vi "Supported .NET colors.vi"() -> (0 "Color Names":T1[](array[typedef]), 2 "Colors":u32[](array[numeric]))   [LabVIEW 2021, in "Rich Text Box.lvlib"]
uses:
  Rich Text Box.lvlib
  Text Colors.ctl
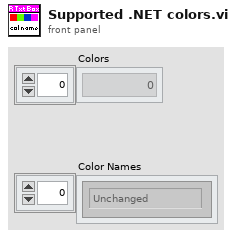
[diagram p1: front panel]
types:
  T1 = typedef "Rich Text Box.lvlib/Text Colors.ctl" = enum16{"Unchanged", "Black", "Blue", "Cyan", "Maroon", "Gray", "Violet", "Green", "Light Green", "Orange", "Yellow", "Magenta", "Red", "White"}
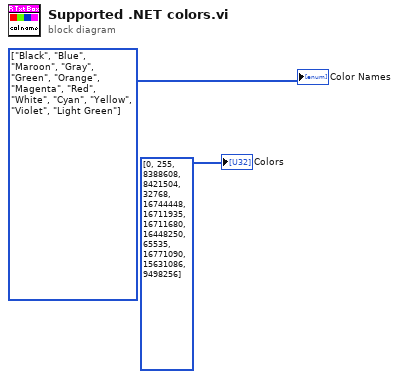
[diagram p0: block diagram]
diagram:
  w2 = T1[] [enum."Black", enum."Blue", enum."Maroon", enum."Gray", enum."Green", enum."Orange", enum."Magenta", enum."Red", enum."White", enum."Cyan", enum."Yellow", enum."Violet", enum."Light Green"] items=["Unchanged", "Black", "Blue", "Cyan", "Maroon", "Gray", "Violet", "Green", "Light Green", "Orange", "Yellow", "Magenta", "Red", "White"] ("Supported Text Color")
  "Color Names" <- w2
  "Colors" <- u32[] [0, 255, 8388608, 8421504, 32768, 16744448, 16711935, 16711680, 16448250, 65535, 16771090, 15631086, 9498256]
